vi "实验封面路径.vi"() -> ()   [LabVIEW 2013]
panel:
  in  "实验封面路径":path=path "C:/Users/Xiang MU/Desktop/实验文件夹/DR96-16-6203-020/GV1/GV1-表格.txt"
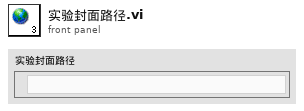
[diagram p1: front panel]
diagram:
